vi "Disconnect.vi"(8 "error in (no error)":errorcluster, 11 "controllers":refnum<k24>[](array[refnum])) -> (0 "error out":errorcluster)   [LabVIEW 2019]
uses:
  C:/Users/patrick/Documents/GitHub/levylabpitt/Aerotech-Delay-Line/lvsrc/Aerotech-Ensemble-LabVIEW/2010-5.6/Bin/Aerotech.Ensemble.dll
  Bin/Aerotech.Ensemble.dll
  C:/Users/patrick/Documents/GitHub/levylabpitt/Aerotech-Delay-Line/lvsrc/Aerotech-Ensemble-LabVIEW/2010-5.6/Bin/Aerotech.Ensemble.LabVIEW.dll
  Bin/Aerotech.Ensemble.LabVIEW.dll
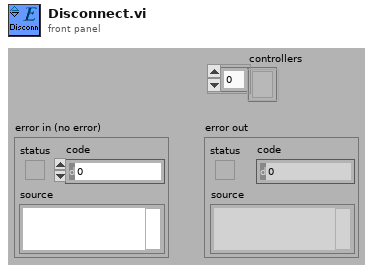
[diagram p1: front panel]
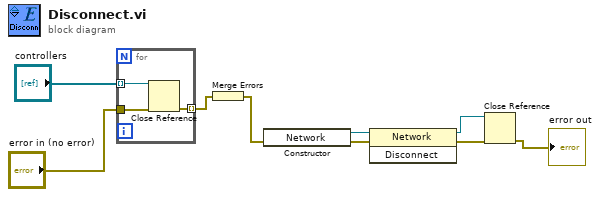
[diagram p0: block diagram]
diagram:
  n1 = for {
    tunnel: "error in (no error)" -> [w12]
    tunnel: [w11] -> w7 mode=indexing
    tunnel: "controllers" -> [w10] mode=indexing
    n2 = Close Reference(reference=w10, error in (no error)=w12) -> (error out=w11:errorcluster)
  }
  n3 = Merge Errors(w7) -> (w1:errorcluster)
  n4 = constructor class="Network"(error in=w1) -> (reference out=w2:refnum<k24>, error out=w6:errorcluster)  [unwired: 2 in, 1 out]
  n5 = invoke class="Network" method="Disconnect"(reference=w2, error in=w6) -> (reference out=w3:refnum<k24>, error out=w5:errorcluster)  [unwired: 1 in, 1 out]
  n6 = Close Reference(reference=w3, error in (no error)=w5) -> (error out=→"error out":errorcluster)
